vi "Parameters.vi"() -> ()   [LabVIEW 2021]
uses:
  Parameters/GetAxisParameterString.vi
  Parameters/GetAxisParameterDouble.vi
  Parameters/SetAxisParameterDouble.vi
  Parameters/SetAxisParameterString.vi
  Parameters/GetTaskParameterDouble.vi
  Parameters/SetTaskParameterDouble.vi
  Parameters/GetSystemParameterDouble.vi
  Parameters/SetSystemParameterDouble.vi
panel:
  out "RadiusCorrectionThreshold":dbl
  out "Error Status":bool
  in  "Send":bool caption="Save"
  out "error out":errorcluster
  in  "Parameter File":path=path "C:/A3200.prma" caption="File Name and Path"
  out "UnitsName":string
  out "InPositionDistance":dbl
  out "SecondaryUnitsScaleFactor":i32
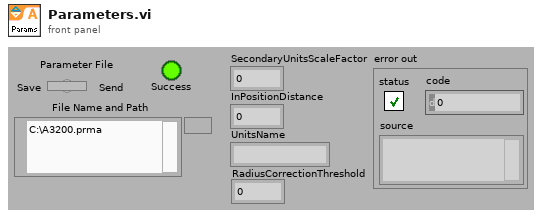
[diagram p1: front panel]
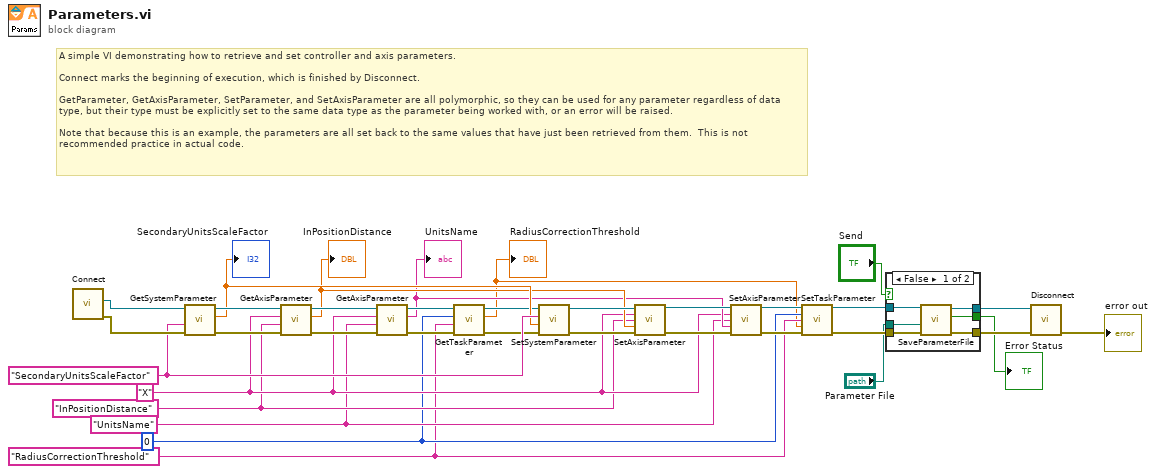
[diagram p0: block diagram]
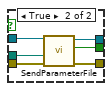
[diagram p2: hidden frame]
diagram:
  w3 = "RadiusCorrectionThreshold" ("paramName")
  w4 = 0 ("Task Number")
  w18 = "X" ("axisName")
  w16 = "UnitsName" ("paramName")
  w17 = "InPositionDistance" ("paramName")
  w22 = "SecondaryUnitsScaleFactor" ("paramName")
  # "A simple VI demonstrating how to retrieve and set controller and axis parameters.\n\nConnect marks the beginning of execution, which is finished by Disconnect.\n\nGetParameter, GetAxisParameter, SetParameter, and SetAxisParameter are all polymorphic, so they can be used for any parameter regardless of data type, but their type must be explicitly set to the same data type as the parameter being worked with, or an error will be raised.\n\nNote that because this is an example, the parameters are all set back to the same values that have just been retrieved from them.  This is not recommended practice in actual code."
  n1 = call "Connect.vi"() -> ("error out"=w32:errorcluster, "controller"=w33:refnum<k24>)  [unwired: 10 in]
  n2 = call-poly "GetSystemParameter.vi"("error in (no error)"=w32, "Parameter Name"=w22, "controller in"=w33) -> ("error out"=w30:errorcluster, "value"=w21:dbl, "controller out"=w31:refnum<k24>)  [unwired: 6 in]
  "SecondaryUnitsScaleFactor" <- w21
  n3 = call-poly "GetAxisParameter.vi"("error in (no error)"=w30, "Parameter Name"=w17, "axis name"=w18, "controller in"=w31) -> ("error out"=w28:errorcluster, "value"=w20:dbl, "controller out"=w29:refnum<k24>)  [unwired: 5 in]
  "InPositionDistance" <- w20
  n4 = call-poly "GetAxisParameter.vi"("error in (no error)"=w28, "Parameter Name"=w16, "axis name"=w18, "controller in"=w29) -> ("error out"=w7:errorcluster, "value"=w19:string, "controller out"=w27:refnum<k24>)  [unwired: 5 in]
  "UnitsName" <- w19
  n5 = call-poly "GetTaskParameter.vi"("error in (no error)"=w7, "Parameter Name"=w3, "taskId"=w4, "controller in"=w27) -> ("error out"=w6:errorcluster, "value"=w2:dbl, "controller out"=w8:refnum<k24>)  [unwired: 5 in]
  "RadiusCorrectionThreshold" <- w2
  n6 = call-poly "SetSystemParameter.vi"("error in (no error)"=w6, "value"=w21, "Parameter Name"=w22, "controller in"=w8) -> ("error out"=w23:errorcluster, "controller out"=w26:refnum<k24>)  [unwired: 4 in]
  n7 = call-poly "SetAxisParameter.vi"("Controller In"=w26, "axisName"=w18, "Parameter Name"=w17, "value"=w20, "error in (no error)"=w23) -> ("Controller Out"=w25:refnum<k24>, "error out"=w24:errorcluster)  [unwired: 9 in]
  n8 = call-poly "SetAxisParameter.vi"("Controller In"=w25, "axisName"=w18, "Parameter Name"=w16, "value"=w19, "error in (no error)"=w24) -> ("Controller Out"=w13:refnum<k24>, "error out"=w15:errorcluster)  [unwired: 9 in]
  n9 = call-poly "SetTaskParameter.vi"("Controller In"=w13, "taskId"=w4, "Parameter Name"=w3, "value"=w2) -> ("Controller Out"=w5:refnum<k24>)  [unwired: 10 in, 1 out]
  n10 = case shown="False" "Send" {
    tunnel: w15 -> [w39 w45]
    tunnel: [w38 w44] -> w14
    tunnel: w5 -> [w36 w43]
    tunnel: "Parameter File" -> [w37 w42]
    tunnel: [w35 w41] -> w9
    tunnel: [w34 w40] -> w1
    frame False {
      n11 = call "SaveParameterFile.vi"("error in (no error)"=w39, "Parameter File path and name"=w37, "controller in"=w36) -> ("error out"=w38:errorcluster, "Error Status"=w35:bool, "controller out"=w34:refnum<k24>)  [unwired: 6 in]
    }
    frame True {
      n12 = call "SendParameterFile.vi"("error in (no error)"=w45, "Parameter File path and name"=w42, "controller in"=w43) -> ("error out"=w44:errorcluster, "Error Status"=w41:bool, "controller out"=w40:refnum<k24>)  [unwired: 6 in]
    }
  }
  "Error Status" <- w9
  n13 = call "Disconnect.vi"("error in (no error)"=w14, "controller"=w1) -> ("error out"=→"error out":errorcluster)  [unwired: 9 in]
